vi "Open Simulation.vi"   [LabVIEW 2013]
doc: "This VI opens the AFM Simulator."
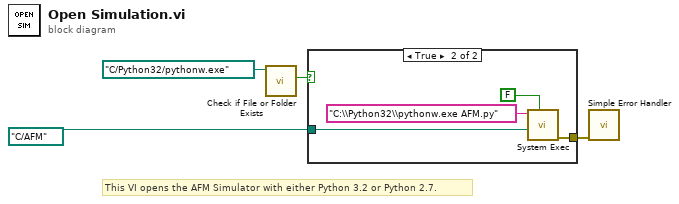
[diagram p0: block diagram]
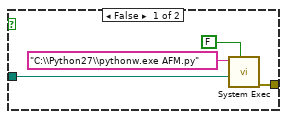
[diagram p2: hidden frame]
diagram:
  # "This VI opens the AFM Simulator with either Python 3.2 or Python 2.7."
  n1 = call <vilib>:"Check if File or Folder Exists.vi"("path"=path "C:/Python32/pythonw.exe") -> ("file or folder exists?"=w3:bool)  [unwired: 8 in, 2 out]
  n2 = case shown="True" w3 {
    tunnel: [w6 w10] -> w2
    tunnel: path "C:/AFM" -> [w5 w9]
    frame False {
      n3 = call <vilib>:"System Exec.vi"("wait until completion? (T)"=FALSE, "working directory"=w5, "command line"="C:\\Python27\\pythonw.exe AFM.py") -> ("error out"=w6:errorcluster)  [unwired: 5 in, 3 out]
    }
    frame True {
      n4 = call <vilib>:"System Exec.vi"("wait until completion? (T)"=FALSE, "working directory"=w9, "command line"="C:\\Python32\\pythonw.exe AFM.py") -> ("error out"=w10:errorcluster)  [unwired: 5 in, 3 out]
    }
  }
  n5 = call <vilib>:"Simple Error Handler.vi"("error in (no error)"=w2) -> ()  [unwired: 4 in, 5 out]
